vi "GetType.vi"(0 "reference in":refnum<class "DI.lvclass">) -> (4 "reference out":refnum<class "DI.lvclass">, 6 "obj_type":T1)   [LabVIEW 2019, in "DI.lvclass"]
uses:
  DI.lvclass
  Logger_class/ObjType.ctl
  Logger_class/Logger.lvclass
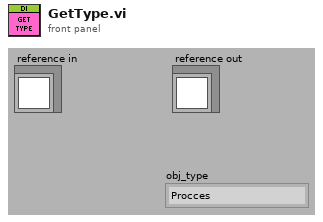
[diagram p1: front panel]
types:
  T1 = typedef "Logger.lvclass/ObjType.ctl" = enum16{"Procces", "Device", "Signal", "DI", "DO", "DA", "AI", "AO", "AA"}
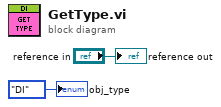
[diagram p0: block diagram]
diagram:
  "reference out" <- "reference in"
  "obj_type" <- ObjType."DI" ("obj_type")
